vi "Read Buffer Size.vi"(8 "error in (no error)":errorcluster, 11 "Node Ptr":T1 format="%.0x") -> (0 "error out":errorcluster, 2 "Buffer Size":u32, 3 "Node Ptr out":T1 format="%.0x")   [LabVIEW 2019, in "UDP-Custom-Device System Explorer.lvlib" / "Buffered Data Packet.lvlib"]
uses:
  Buffered Data Packet.lvlib
  <vilib>/NI VeriStand/Custom Device API/Custom Device Item Ref.ctl
  Shared/Constants.vi
  <vilib>/NI VeriStand/Custom Device API/Get Item Property (U32).vi
  <vilib>/NI VeriStand/Custom Device API/Custom Device API.lvlib
  Shared/UDP-Custom-Device Shared.lvlib
  UDP-Custom-Device System Explorer.lvlib
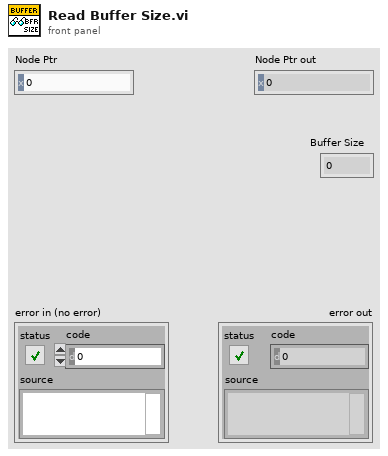
[diagram p1: front panel]
types:
  T1 = typedef "Custom Device API.lvlib/Custom Device Item Ref.ctl" = u64
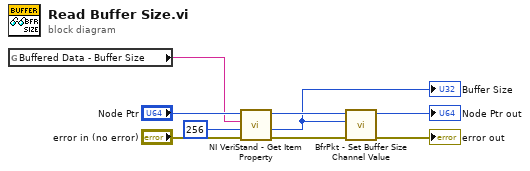
[diagram p0: block diagram]
diagram:
  n1 = global read "Constants.vi" "Buffered Data - Buffer Size"() -> (w7:string)
  n2 = call-poly <vilib>:"NI VeriStand - Get Item Property.vi"("error in (no error)"="error in (no error)", "Default Value"=u32 256, "Property Name"=w7, "Item Ref in"="Node Ptr") -> ("error out"=w2:errorcluster, "Value"=w3:u32, "Item Ref out"=w5:T1)  [unwired: 4 in, 1 out]
  "Buffer Size" <- w3
  n3 = call "BfrPkt - Set Buffer Size Channel Value.vi"("error in (no error)"=w2, "Buffer Size"=w3, "Node Ptr"=w5) -> ("error out"=→"error out":errorcluster, "Node Ptr out"=→"Node Ptr out":T1)  [unwired: 7 in]
